vi "Setup Path.vi"(0 "Path in":refnum<class "Path.lvclass">, 5 "TSM Context":T1, 7 "Path Callbacks":refnum<vi>[](array[refnum]), 11 "error in":errorcluster) -> (4 "Path out":refnum<class "Path.lvclass">, 15 "error out":errorcluster)   [LabVIEW 2023, in "RFCalAndFixtureCharact.Common.lvlib"]
uses:
  RFCalAndFixtureCharact.Common.lvlib
  Base Classes/Path/Path.lvclass
  <vilib>/NI_TestStand_SemiconductorModule/NI_TestStand_Semiconductor_Module.lvlibp/PinMap/General/SemiconductorModuleContext.ctl
  <vilib>/NI_TestStand_SemiconductorModule/NI_TestStand_Semiconductor_Module.lvlibp
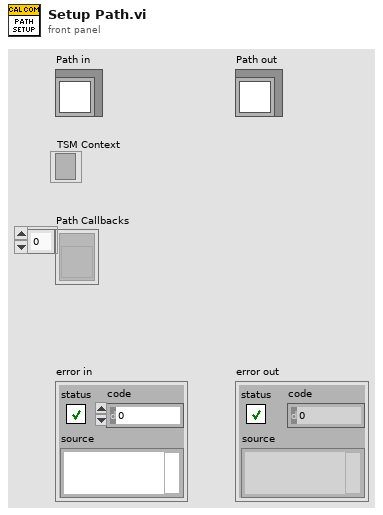
[diagram p1: front panel]
types:
  T1 = typedef "NI_TestStand_Semiconductor_Module.lvlibp/SemiconductorModuleContext.ctl" = refnum<k7>
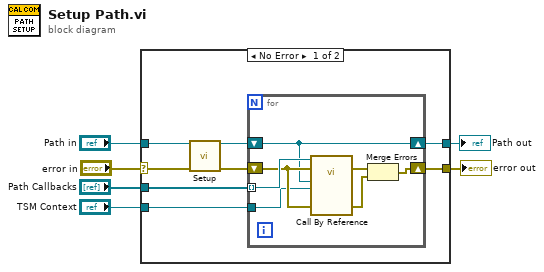
[diagram p0: block diagram]
diagram:
  n1 = case shown="No Error" "error in" {
    selector: "error in" -> [w14 w23]
    tunnel: "Path in" -> [w13 w22]
    tunnel: [w12 w23] -> w4
    tunnel: [w10 w22] -> w3
    tunnel: "TSM Context" -> [w9 _]
    tunnel: "Path Callbacks" -> [w8 _]
    frame No Error {
      n2 = call-dynamic "Setup.vi"("Path in"=w13, "error in (no error)"=w14) -> ("Path out"=w11:refnum<class "Path.lvclass">, "error out"=w7:errorcluster)  [unwired: 12 in]
      n3 = for {
        shift-right: [w19] -> w12
        shift-left: w7 -> [w17]
        tunnel: w8 -> [w21] mode=indexing
        shift-right: [w16] -> w10
        shift-left: w11 -> [w16]
        tunnel: w9 -> [w15]
        n4 = call-by-ref "?"(reference=w21, error in=w17, "RFCalAndFixtureCharact.Common.lvlib:Path.lvclass"=w16, "TSM Context"=w15, "error in"=w17) -> (error out=w20:errorcluster, 15:"error out"=w18:errorcluster)  [unwired: 12 in, 1 out]
        n5 = Merge Errors(w20, w18) -> (w19:errorcluster)
      }
    }
    frame Error {
    }
  }
  "error out" <- w4
  "Path out" <- w3
